vi "Configure DID & PID Dialog.vi"(6 "Signals":T1[](array[typedef]) {"Byte Order" items=["Little Endian", "Big Endian"]; "Data Type" items=["Signed", "Unsigned", "IEEE Float"]}, 7 "Show Name&ID":bool=TRUE, 8 "error in (no error)":errorcluster, 9 "ID":u16=1 min=1 format="%.0x", 10 "Existing PIDs":string[](array[string]), 11 "Name":string) -> (0 "error out":errorcluster, 1 "ID out":u16=1 min=1 format="%.0x", 2 "Cancel PID?":bool, 3 "Name out":string, 4 "Signals out":T1[](array[typedef]) {"Byte Order" items=["Little Endian", "Big Endian"]; "Data Type" items=["Signed", "Unsigned", "IEEE Float"]})   [LabVIEW 2015, in "Diagnostics Addon System Explorer.lvlib"]
uses:
  Diagnostics Addon System Explorer.lvlib
  Shared/Types/Signal Parameters.ctl
  <vilib>/NI/AMC/Create Single Message.vi
  <vilib>/NI/AMC/Update Message Routing Info.vi
  <vilib>/NI/AMC/Read Termination Message.vi
  <vilib>/NI/AMC/Send Message.vi
  <vilib>/NI/AMC/Globals.vi
  Shared/Diagnostics Addon Shared.lvlib
  <vilib>/NI/AMC/AMC.lvlib
panel:
  in  "Endian":u8(ring) items=["Little", "Big"]
  in  "Datatype":u8(ring)=1 items=["Signed", "Unsigned", "Float"]
  in  "Remove":bool
  in  "Add":bool
  in  "Cancel PID":bool
  in  "Apply":bool
  in  "Cancel":bool
  in  "OK":bool
  in  "Maximum":dbl=255.0
  in  "Minimum":dbl
  in  "Offset":dbl
  in  "Factor":dbl=1.0
  in  "Length":u8=8
  in  "Start Bit":u8
  in  "Signal Name":string
  in  "Signals":i32(listbox)
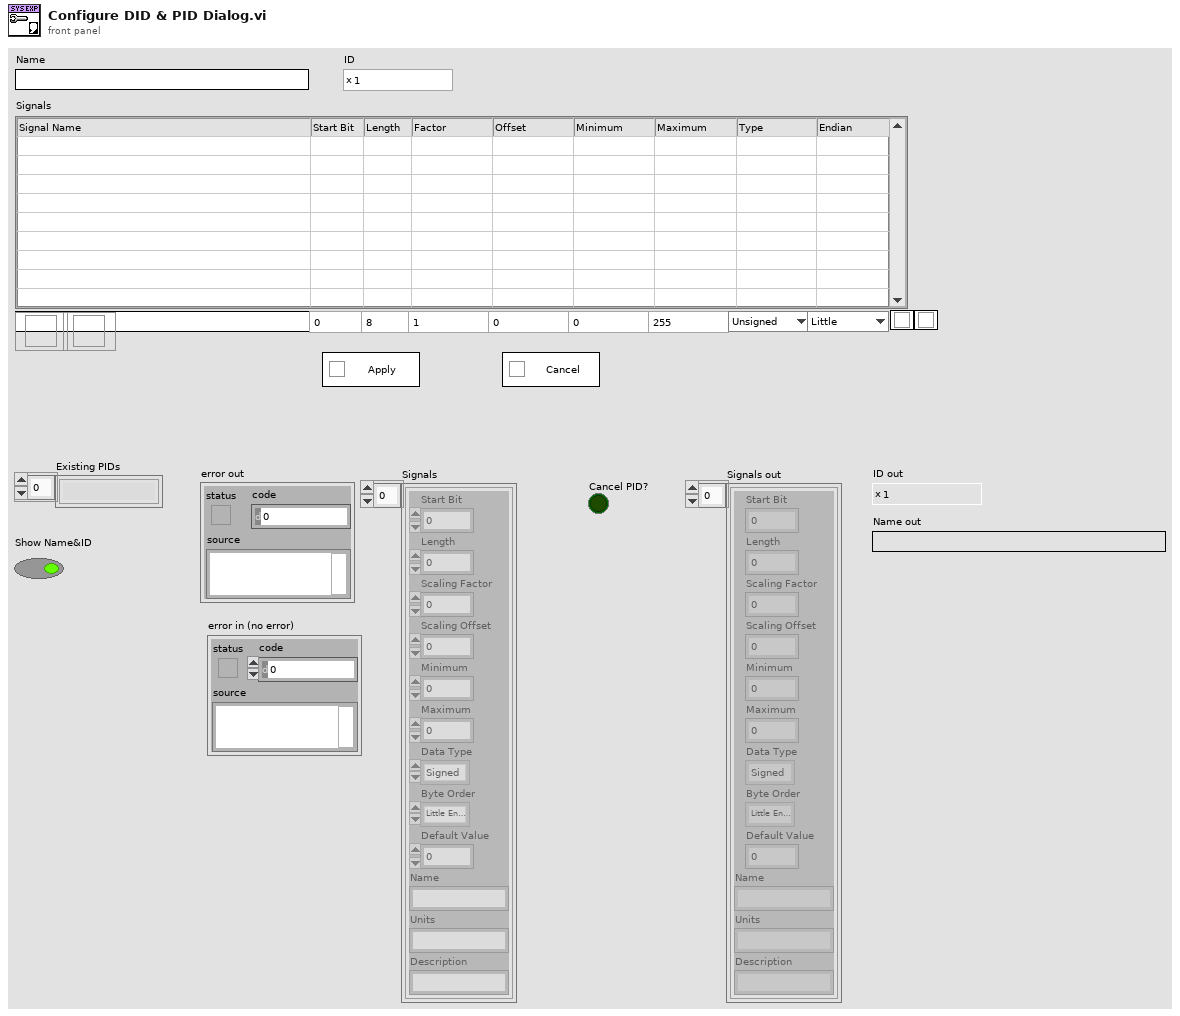
[diagram p1: front panel]
types:
  T1 = typedef "Diagnostics Addon Shared.lvlib/Signal Parameters.ctl" = cluster{"Start Bit":u8, "Length":u8, "Scaling Factor":dbl, "Scaling Offset":dbl, "Minimum":dbl, "Maximum":dbl, "Data Type":u32, "Byte Order":u32, "Default Value":dbl, "Name":string, "Units":string, "Description":string}
  T2 = cluster{"NewControlRefs":refnum<vi>[], "Add":refnum<vi>, "Listbox":refnum<vi>, "Remove":refnum<vi>, "Apply":refnum<vi>, "Cancel PID":refnum<vi>}
  T3 = typedef "AMC.lvlib/Message Queue.ctl" = refnum<queue>
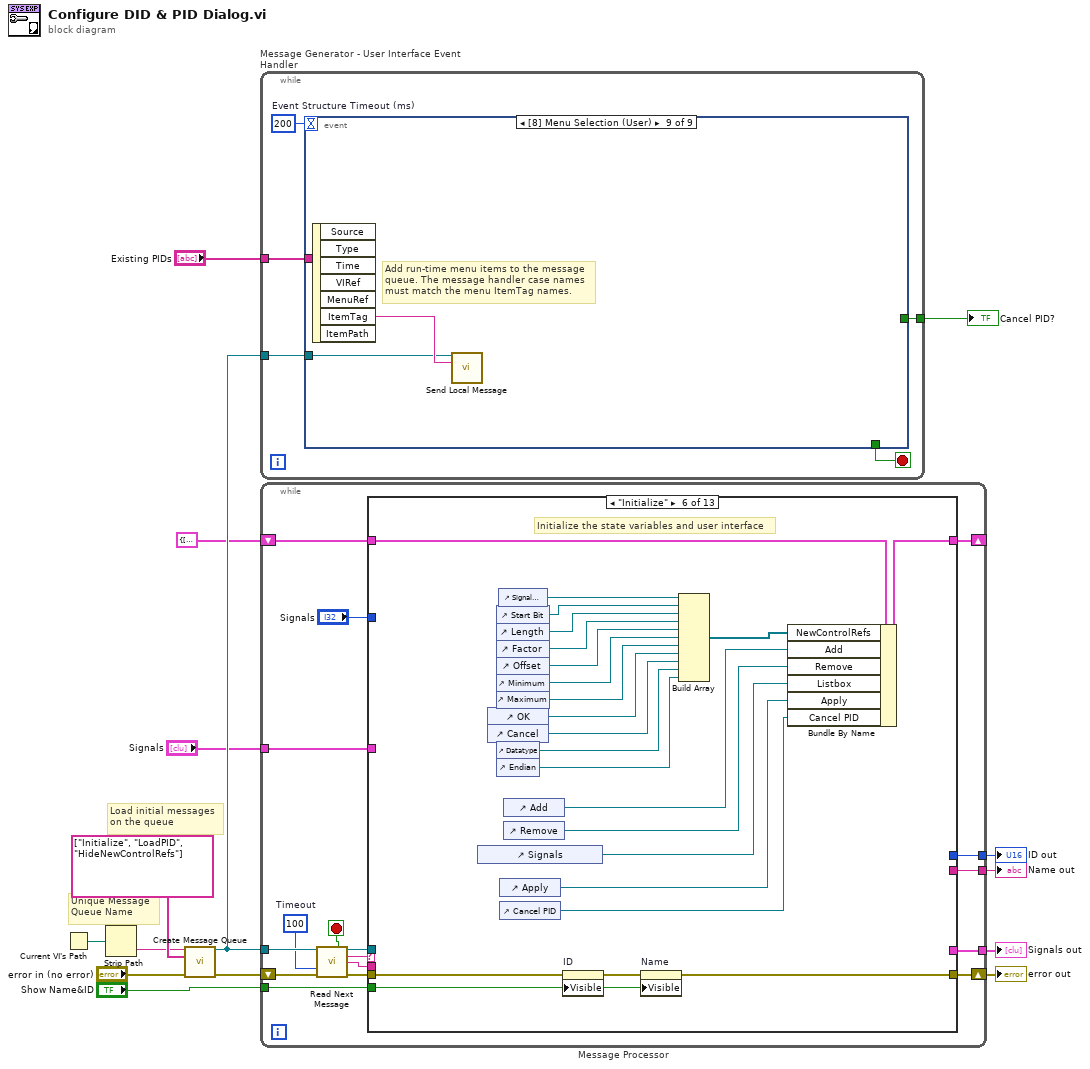
[diagram p0: block diagram]
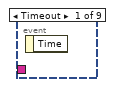
[diagram p2: hidden frame]
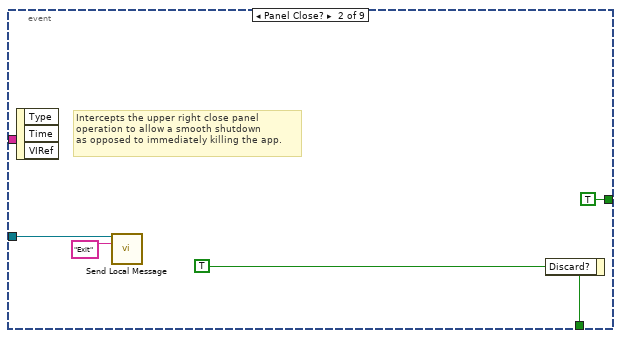
[diagram p3: hidden frame]
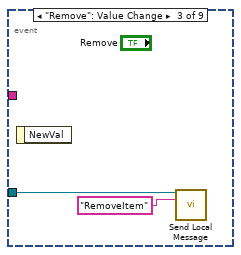
[diagram p4: hidden frame]
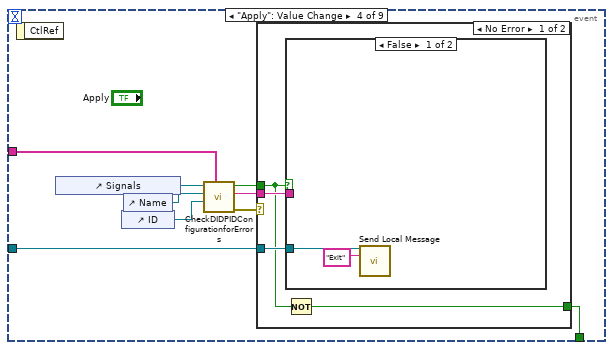
[diagram p5: hidden frame]
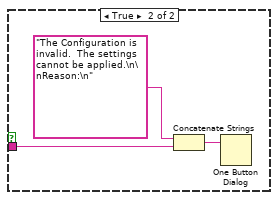
[diagram p6: hidden frame]
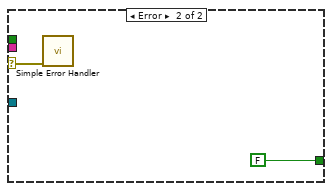
[diagram p7: hidden frame]
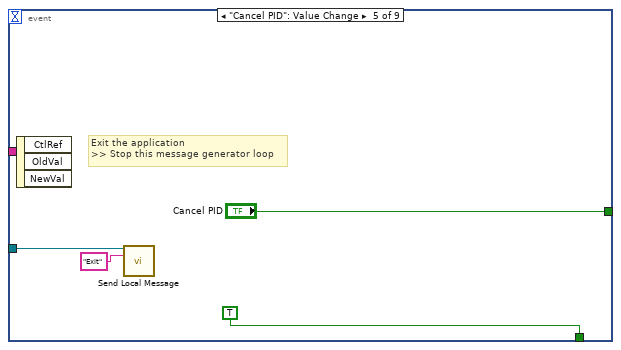
[diagram p8: hidden frame]
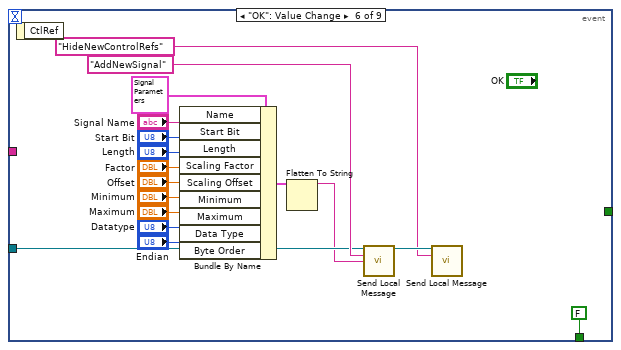
[diagram p9: hidden frame]
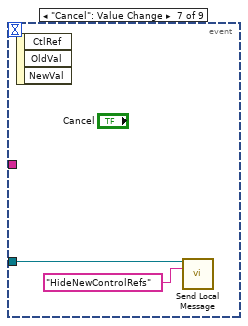
[diagram p10: hidden frame]
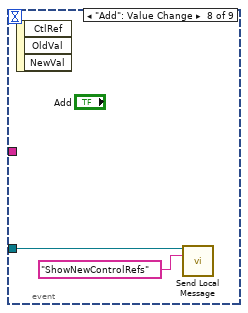
[diagram p11: hidden frame]
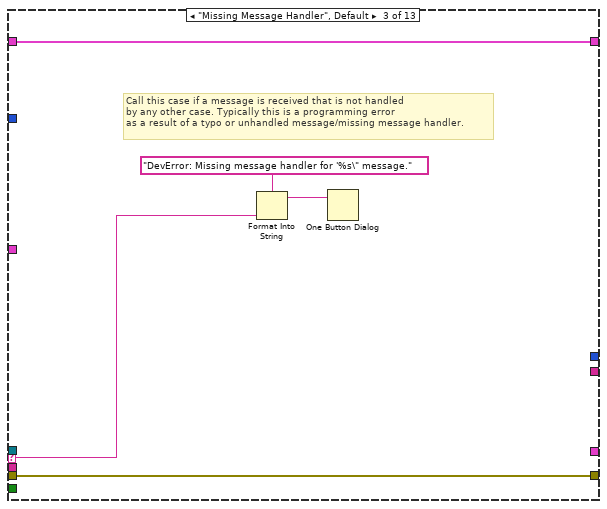
[diagram p14: hidden frame]
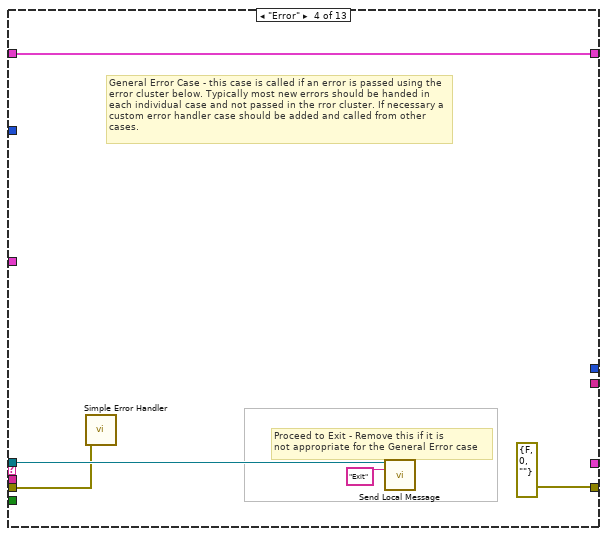
[diagram p15: hidden frame]
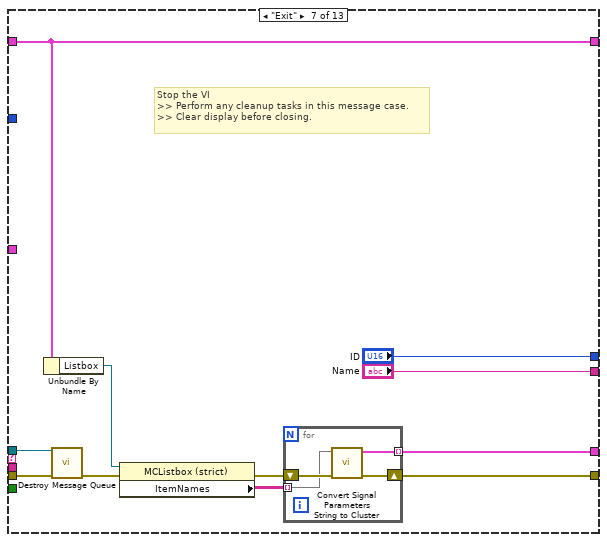
[diagram p17: hidden frame]
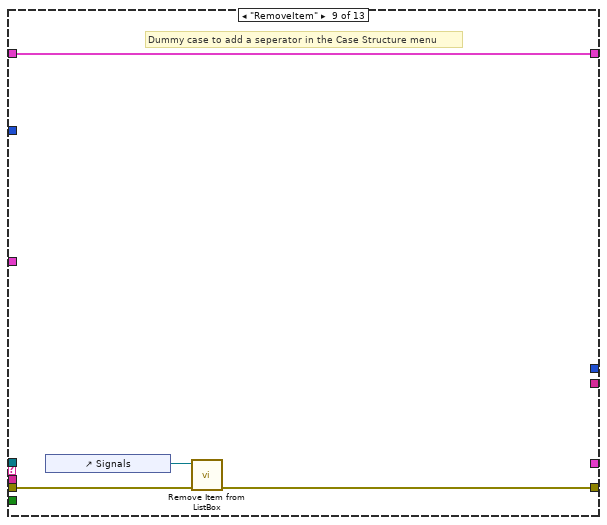
[diagram p19: hidden frame]
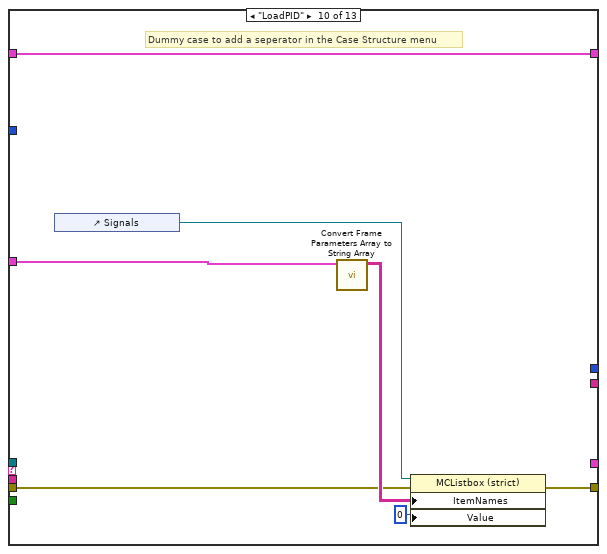
[diagram p20: hidden frame]
diagram:
  # "Unique Message\nQueue Name"
  # "Load initial messages\non the queue"
  n1 = Current VI's Path() -> (path=w11:path)
  n2 = Strip Path(path=w11) -> (name=w14:string)  [unwired: 1 out]
  n3 = call <vilib>:"Create Message Queue.vi"("message queue name"=w14, "initial message names"=string[] ["Initialize", "LoadPID", "HideNewControlRefs"], "error in"="error in (no error)") -> ("message queue out"=w13:T3, "error out"=w12:errorcluster)  [unwired: 11 in]
  n4 = while "Message Generator - User Interface Event Handler" {
    tunnel: w13 -> [w18]
    tunnel: [w17] -> w9
    tunnel: "Existing PIDs" -> [w16]
    stop <- w19 stop-if-true
    w20 = 200  # Event Structure Timeout (ms)
    n5 = event shown="[8] Menu Selection (User)" {
      selector: _ -> [_ _ _ _ _ _ _ _ _]
      dyn-events: _ -> [_ _ _ _ _ _ _ _ _]
      timeout: w20 -> [_ _ _ _ _ _ _ _ _]
      tunnel: [_ w24 _ w27 TRUE ("Discard?") FALSE ("Discard?") _ _ _] -> w19
      tunnel: w18 -> [_ w22 w25 w33 w48 w65 w68 w70 w72]
      tunnel: [_ TRUE ("Cancel PID") _ _ "Cancel PID" _ _ _ _] -> w17
      tunnel: w16 -> [_ _ _ w30 _ _ _ _ _]
      event Timeout {
        n6 = event-data() -> ()  [unwired: 2 out]
      }
      event Panel Close? {
        w24 = TRUE ("Discard?")
        # "Intercepts the upper right close panel\noperation to allow a smooth shutdown\nas opposed to immediately killing the app."
        n7 = event-data() -> ()  [unwired: 4 out]
        n8 = call <vilib>:"Send Local Message.vi"("message queue in"=w22, "message name"="Exit") -> ()  [unwired: 11 in, 3 out]
        n9 = event-data("Discard?"=w24) -> ()  [unwired: 1 in, 1 out]
      }
      event "Remove": Value Change {
        n10 = event-data() -> ()  [unwired: 2 out]
        n11 = call <vilib>:"Send Local Message.vi"("message queue in"=w25, "message name"="RemoveItem") -> ()  [unwired: 11 in, 3 out]
      }
      event "Apply": Value Change {
        n12 = event-data() -> ()  [unwired: 2 out]
        n13 = control-ref of="Signals"() -> (w35:refnum<vi>)
        n14 = control-ref of="ID"() -> (w31:refnum<vi>)
        n15 = control-ref of="Name"() -> (w32:refnum<vi>)
        n16 = call "CheckDIDPIDConfigurationforErrors.vi"("Existing PIDs"=w30, "ID"=w31, "Name"=w32, "Listbox"=w35) -> ("error out"=w28:errorcluster, "Error Type"=w29:string, "Error?"=w34:bool)  [unwired: 5 in]
        n17 = case shown="No Error" w28 {
          selector: w28 -> [_ w46]
          tunnel: w34 -> [w37 _]
          tunnel: w33 -> [w39 _]
          tunnel: w29 -> [w38 _]
          tunnel: [w36 FALSE] -> w27
          frame No Error {
            n18 = case shown="False" w37 {
              tunnel: w39 -> [w41 _]
              tunnel: w38 -> [_ w44]
              frame False {
                n19 = call <vilib>:"Send Local Message.vi"("message queue in"=w41, "message name"="Exit" ("Message Name")) -> ()  [unwired: 11 in, 3 out]
              }
              frame True {
                n20 = Concatenate Strings("The Configuration is invalid.  The settings cannot be applied.\n\nReason:\n" ("message"), w44) -> (w42:string)
                n21 = One Button Dialog(message=w42) -> ()  [unwired: 1 in, 1 out]
              }
            }
            n22 = Not(x=w37) -> (.not. x?=w36:bool)
          }
          frame Error {
            n23 = call <vilib>:"Simple Error Handler.vi"("error in (no error)"=w46) -> ()  [unwired: 4 in, 5 out]
          }
        }
      }
      event "Cancel PID": Value Change {
        # "Exit the application\n>> Stop this message generator loop"
        n24 = event-data() -> ()  [unwired: 4 out]
        n25 = call <vilib>:"Send Local Message.vi"("message queue in"=w48, "message name"="Exit") -> ()  [unwired: 11 in, 3 out]
      }
      event "OK": Value Change {
        n26 = event-data() -> ()  [unwired: 2 out]
        n27 = Bundle By Name(cluster=T1 {"Start Bit"=0, "Length"=0, "Scaling Factor"=0.0, "Scaling Offset"=0.0, "Minimum"=0.0, "Maximum"=0.0, "Data Type"=0, "Byte Order"=0, "Default Value"=0.0, "Name"="", "Units"="", "Description"=""} ("Signal Parameters"), "Name"="Signal Name", "Start Bit"="Start Bit", "Length"="Length", "Scaling Factor"="Factor", "Scaling Offset"="Offset", "Minimum"="Minimum", "Maximum"="Maximum", "Data Type"="Datatype", "Byte Order"="Endian") -> (w56:T1)
        n28 = Flatten To String(anything=w56) -> (data string=w55:string)  [unwired: 3 in, 2 out]
        n29 = call <vilib>:"Send Local Message.vi"("message queue in"=w65, "message name"="AddNewSignal", "message value"=w55) -> ("message queue out"=w54:T3)  [unwired: 10 in, 2 out]
        n30 = call <vilib>:"Send Local Message.vi"("message queue in"=w54, "message name"="HideNewControlRefs" ("Message Name")) -> ()  [unwired: 11 in, 3 out]
      }
      event "Cancel": Value Change {
        n31 = event-data() -> ()  [unwired: 4 out]
        n32 = call <vilib>:"Send Local Message.vi"("message queue in"=w68, "message name"="HideNewControlRefs" ("Message Name")) -> ()  [unwired: 11 in, 3 out]
      }
      event "Add": Value Change {
        n33 = event-data() -> ()  [unwired: 4 out]
        n34 = call <vilib>:"Send Local Message.vi"("message queue in"=w70, "message name"="ShowNewControlRefs" ("Message Name")) -> ()  [unwired: 11 in, 3 out]
      }
      event Menu Selection (User) {
        # "Add run-time menu items to the message\nqueue. The message handler case names must match the menu ItemTag names."
        n35 = event-data() -> ("ItemTag"=w73:string)  [unwired: 7 out]
        n36 = call <vilib>:"Send Local Message.vi"("message queue in"=w72, "message name"=w73) -> ()  [unwired: 11 in, 3 out]
      }
    }
  }
  "Cancel PID?" <- w9
  n37 = while "Message Processor" {
    shift-left: w12 -> [w84]
    shift-right: [w88] -> w7
    tunnel: w13 -> [w85]
    shift-left: T2 {"NewControlRefs"=[], "Add"=refnum, "Listbox"=refnum, "Remove"=refnum, "Apply"=refnum, "Cancel PID"=refnum} ("State Variables") -> [w90]
    shift-right: [w89] -> _
    tunnel: "Signals" -> [w78]
    tunnel: [w77] -> w4
    tunnel: [w76] -> w3
    tunnel: [w75] -> w2
    tunnel: "Show Name&ID" -> [w74]
    stop <- w87 stop-if-true
    w82 = 100  # Timeout
    n38 = call <vilib>:"Read Next Message.vi"("message queue in"=w85, "timeout (1 ms)"=w82, "error in"=w84) -> ("exit process?"=w87:bool, "message queue out"=w86:T3, "message name"=w81:string, "message value"=w80:string, "error out"=w83:errorcluster)  [unwired: 5 in, 3 out]
    n39 = case shown="\"Initialize\"" w81 {
      selector: w81 -> [_ _ w97 _ _ _ _ _ _ _ _ _ _]
      tunnel: [w92 w94 w99 w104 w106 w118 w138 w146 w150 w157 w163 w180 w194] -> w89
      tunnel: w90 -> [w92 w94 w99 w104 w106 w119 w138 w146 w150 w157 w163 w180 w194]
      tunnel: w86 -> [_ _ _ w102 _ _ w139 _ _ _ _ _ _]
      tunnel: w83 -> [w91 w93 w98 w100 w105 w109 w140 w145 w148 w151 w166 w179 w193]
      tunnel: [w91 w93 w98 errorcluster {"status"=FALSE, "code"=0, "source"=""} ("error out") w105 w108 w133 w145 w147 w154 w160 w169 w184] -> w88
      tunnel: w80 -> [_ _ _ _ _ _ _ _ _ _ w165 _ _]
      tunnel: "Signals" -> [_ _ _ _ _ _ _ _ _ _ _ _ _]
      tunnel: w78 -> [_ _ _ _ _ _ _ _ _ w152 _ _ _]
      tunnel: [_ _ _ _ _ _ w132 _ _ _ _ _ _] -> w77
      tunnel: [_ _ _ _ _ _ "Name" _ _ _ _ _ _] -> w76
      tunnel: [_ _ _ _ _ _ "ID" _ _ _ _ _ _] -> w75
      tunnel: w74 -> [_ _ _ _ _ w107 _ _ _ _ _ _ _]
      frame "---------- Framework Operations ----------" {
        # "Dummy case to add a seperator in the Case Structure menu"
      }
      frame "", "Idle" {
        # "Idle Case - this case is called after a Timeout on the Get Next Message from Queue VI, if no new messages are present on the queue. This case can be used for housekeeping tasks such as updating the UI."
      }
      frame "Missing Message Handler", Default {
        # "Call this case if a message is received that is not handled \nby any other case. Typically this is a programming error\nas a result of a typo or unhandled message/missing message handler."
        n40 = Format Into String(format string="DevError: Missing message handler for '%s\" message." ("message"), w97) -> (resulting string=w95:string)  [unwired: 2 in, 1 out]
        n41 = One Button Dialog(message=w95) -> ()  [unwired: 2 out]
      }
      frame "Error" {
        # "Proceed to Exit - Remove this if it is\nnot appropriate for the General Error case"
        # "General Error Case - this case is called if an error is passed using the error cluster below. Typically most new errors should be handed in each individual case and not passed in the rror cluster. If necessary a custom error handler case should be added and called from other cases."
        n42 = call <vilib>:"Simple Error Handler.vi"("error in (no error)"=w100) -> ()  [unwired: 1 in, 8 out]
        n43 = call <vilib>:"Send Local Message.vi"("message queue in"=w102, "message name"="Exit") -> ()  [unwired: 11 in, 3 out]
      }
      frame "---------- Generic Operations ----------" {
        # "Dummy case to add a seperator in the Case Structure menu"
      }
      frame "Initialize" {
        # "Initialize the state variables and user interface"
        n44 = control-ref of="Signals"() -> (w116:refnum<vi>)
        n45 = control-ref of="OK"() -> (w128:refnum<vi>)
        n46 = control-ref of="Cancel"() -> (w129:refnum<vi>)
        n47 = control-ref of="Start Bit"() -> (w122:refnum<vi>)
        n48 = control-ref of="Length"() -> (w123:refnum<vi>)
        n49 = control-ref of="Factor"() -> (w124:refnum<vi>)
        n50 = control-ref of="Offset"() -> (w125:refnum<vi>)
        n51 = control-ref of="Minimum"() -> (w126:refnum<vi>)
        n52 = control-ref of="Maximum"() -> (w127:refnum<vi>)
        n53 = control-ref of="Datatype"() -> (w114:refnum<vi>)
        n54 = control-ref of="Endian"() -> (w113:refnum<vi>)
        n55 = control-ref of="Signal Name"() -> (w121:refnum<vi>)
        n56 = control-ref of="Apply"() -> (w112:refnum<vi>)
        n57 = control-ref of="Cancel PID"() -> (w111:refnum<vi>)
        n58 = control-ref of="Add"() -> (w117:refnum<vi>)
        n59 = control-ref of="Remove"() -> (w115:refnum<vi>)
        n60 = property on="ID" class="DigNum (strict)"(error in=w109, "Visible"=w107) -> (error out=w110:errorcluster)  [unwired: 1 in, 1 out]
        n61 = property on="Name" class="Str"(error in=w110, "Visible"=w107) -> (error out=w108:errorcluster)  [unwired: 1 in, 1 out]
        n62 = Build Array(w121, w122, w123, w124, w125, w126, w127, w128, w129, w114, w113) -> (w120:refnum<vi>[])
        n63 = Bundle By Name(cluster=w119, "NewControlRefs"=w120, "Add"=w117, "Remove"=w115, "Listbox"=w116, "Apply"=w112, "Cancel PID"=w111) -> (w118:T2)
      }
      frame "Exit" {
        # "Stop the VI\n>> Perform any cleanup tasks in this message case.\n>> Clear display before closing."
        n64 = Unbundle By Name(w138) -> ("Listbox"=w137:refnum<vi>)
        n65 = call <vilib>:"Destroy Message Queue.vi"("message queue in"=w139, "error in"=w140) -> ("error out"=w136:errorcluster)  [unwired: 11 in, 2 out]
        n66 = property class="MCListbox (strict)"(reference=w137, error in=w136) -> (error out=w134:errorcluster, "ItemNames"=w135:string[][])  [unwired: 1 out]
        n67 = for {
          shift-right: [w143] -> w133
          shift-left: w134 -> [w144]
          tunnel: w135 -> [w142] mode=indexing
          tunnel: [w141] -> w132 mode=indexing
          n68 = call "Convert Signal Parameters String to Cluster.vi"("error in (no error)"=w144, "Signal Parameters"=w142) -> ("error out"=w143:errorcluster, "Signal Parameters"=w141:T1)  [unwired: 8 in]
        }
      }
      frame "---------- Application Operations ----------" {
        # "Dummy case to add a seperator in the Case Structure menu"
      }
      frame "RemoveItem" {
        # "Dummy case to add a seperator in the Case Structure menu"
        n69 = control-ref of="Signals"() -> (w149:refnum<vi>)
        n70 = call "Remove Item from ListBox.vi"("error in (no error)"=w148, "MulticolumnListbox in"=w149) -> ("error out"=w147:errorcluster)  [unwired: 9 in]
      }
      frame "LoadPID" {
        # "Dummy case to add a seperator in the Case Structure menu"
        n71 = control-ref of="Signals"() -> (w156:refnum<vi>)
        n72 = call "Convert Frame Parameters Array to String Array.vi"("Frame Parameters"=w152) -> ("Frame Parameters"=w153:string[][])  [unwired: 9 in, 1 out]
        n73 = property class="MCListbox (strict)"(reference=w156, error in=w151, "ItemNames"=w153, "Value"=0) -> (error out=w154:errorcluster)  [unwired: 1 out]
      }
      frame "AddNewSignal" {
        # "Dummy case to add a seperator in the Case Structure menu"
        n74 = Unflatten From String(type=T1 {"Start Bit"=0, "Length"=0, "Scaling Factor"=0.0, "Scaling Offset"=0.0, "Minimum"=0.0, "Maximum"=0.0, "Data Type"=0, "Byte Order"=0, "Default Value"=0.0, "Name"="", "Units"="", "Description"=""} ("Signal Parameters"), binary string=w165, error in (no error)=w166) -> (value=w159:T1, error out=w161:errorcluster)  [unwired: 2 in, 1 out]
        n75 = Unbundle By Name(w163) -> ("Listbox"=w162:refnum<vi>)
        n76 = call "Convert Signal Cluster to String Array.vi"("Signal Parameters"=w159) -> ("Array"=w158:string[])  [unwired: 10 in]
        n77 = call "Add Item to Listbox.vi"("error in (no error)"=w161, "Item"=w158, "MulticolumnListbox in"=w162) -> ("error out"=w160:errorcluster)  [unwired: 8 in]
      }
      frame "HideNewControlRefs" {
        w171 = TRUE ("Visible")
        # "Dummy case to add a seperator in the Case Structure menu"
        n78 = Unbundle By Name(w180) -> ("Cancel PID"=w167:refnum<vi>, "Apply"=w168:refnum<vi>, "Remove"=w173:refnum<vi>, "Add"=w175:refnum<vi>, "NewControlRefs"=w178:refnum<vi>[])
        n79 = call "Visible Control References.vi"("error in"=w179, "Visible?"=FALSE, "Control Refs"=w178) -> ("error out"=w176:errorcluster)  [unwired: 8 in]
        n80 = property class="Bool"(reference=w175, error in=w176, "Visible"=w171) -> (error out=w174:errorcluster)  [unwired: 1 out]
        n81 = property class="Bool"(reference=w173, error in=w174, "Visible"=w171) -> (error out=w170:errorcluster)  [unwired: 1 out]
        n82 = property class="Bool"(reference=w168, error in=w170, "Visible"=w171) -> (error out=w172:errorcluster)  [unwired: 1 out]
        n83 = property class="Bool"(reference=w167, error in=w172, "Visible"=w171) -> (error out=w169:errorcluster)  [unwired: 1 out]
      }
      frame "ShowNewControlRefs" {
        w183 = FALSE ("Visible")
        # "Dummy case to add a seperator in the Case Structure menu"
        n84 = Unbundle By Name(w194) -> ("Apply"=w182:refnum<vi>, "Cancel PID"=w181:refnum<vi>, "Remove"=w187:refnum<vi>, "Add"=w189:refnum<vi>, "NewControlRefs"=w192:refnum<vi>[])
        n85 = call "Visible Control References.vi"("error in"=w193, "Visible?"=TRUE, "Control Refs"=w192) -> ("error out"=w190:errorcluster)  [unwired: 8 in]
        n86 = property class="Bool"(reference=w189, error in=w190, "Visible"=w183) -> (error out=w188:errorcluster)  [unwired: 1 out]
        n87 = property class="Bool"(reference=w187, error in=w188, "Visible"=w183) -> (error out=w185:errorcluster)  [unwired: 1 out]
        n88 = property class="Bool"(reference=w181, error in=w185, "Visible"=w183) -> (error out=w186:errorcluster)  [unwired: 1 out]
        n89 = property class="Bool"(reference=w182, error in=w186, "Visible"=w183) -> (error out=w184:errorcluster)  [unwired: 1 out]
      }
    }
  }
  "error out" <- w7
  "Signals out" <- w4
  "ID out" <- w2
  "Name out" <- w3
